vi "IStageOpen.vi"() -> (1 "PRIORLib.IStageOut":refnum<k7>, 2 "error out":errorcluster)   [LabVIEW 2011]
panel:
  in  "PRIORLib.IStage":refnum<k7>
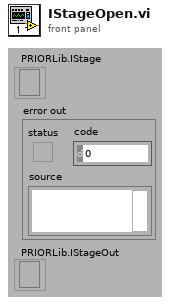
[diagram p1: front panel]
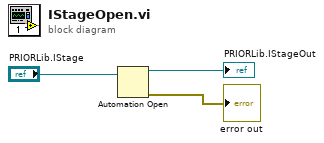
[diagram p0: block diagram]
diagram:
  n1 = Automation Open(Automation Refnum="PRIORLib.IStage") -> (Automation Refnum=→"PRIORLib.IStageOut":refnum<k7>, error out=→"error out":errorcluster)  [unwired: 3 in]
